vi "Coercion Dots.vi"() -> ()   [LabVIEW 2015]
panel:
  out "x+y":i64
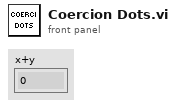
[diagram p1: front panel]
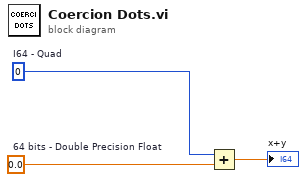
[diagram p0: block diagram]
diagram:
  w1 = 0.0  # 64 bits - Double Precision Float
  w3 = i64 0  # I64 - Quad
  n1 = Add(x=w3, y=w1) -> (x+y=→"x+y":dbl)
